vi "文件保存循环.vi"(8 "错误输入（无错误）":errorcluster, 10 "结束位队列":refnum<queue>, 11 "队列输入":refnum<queue>) -> (3 "总波形图表":waveform(i32)[](graph))   [LabVIEW 2020]
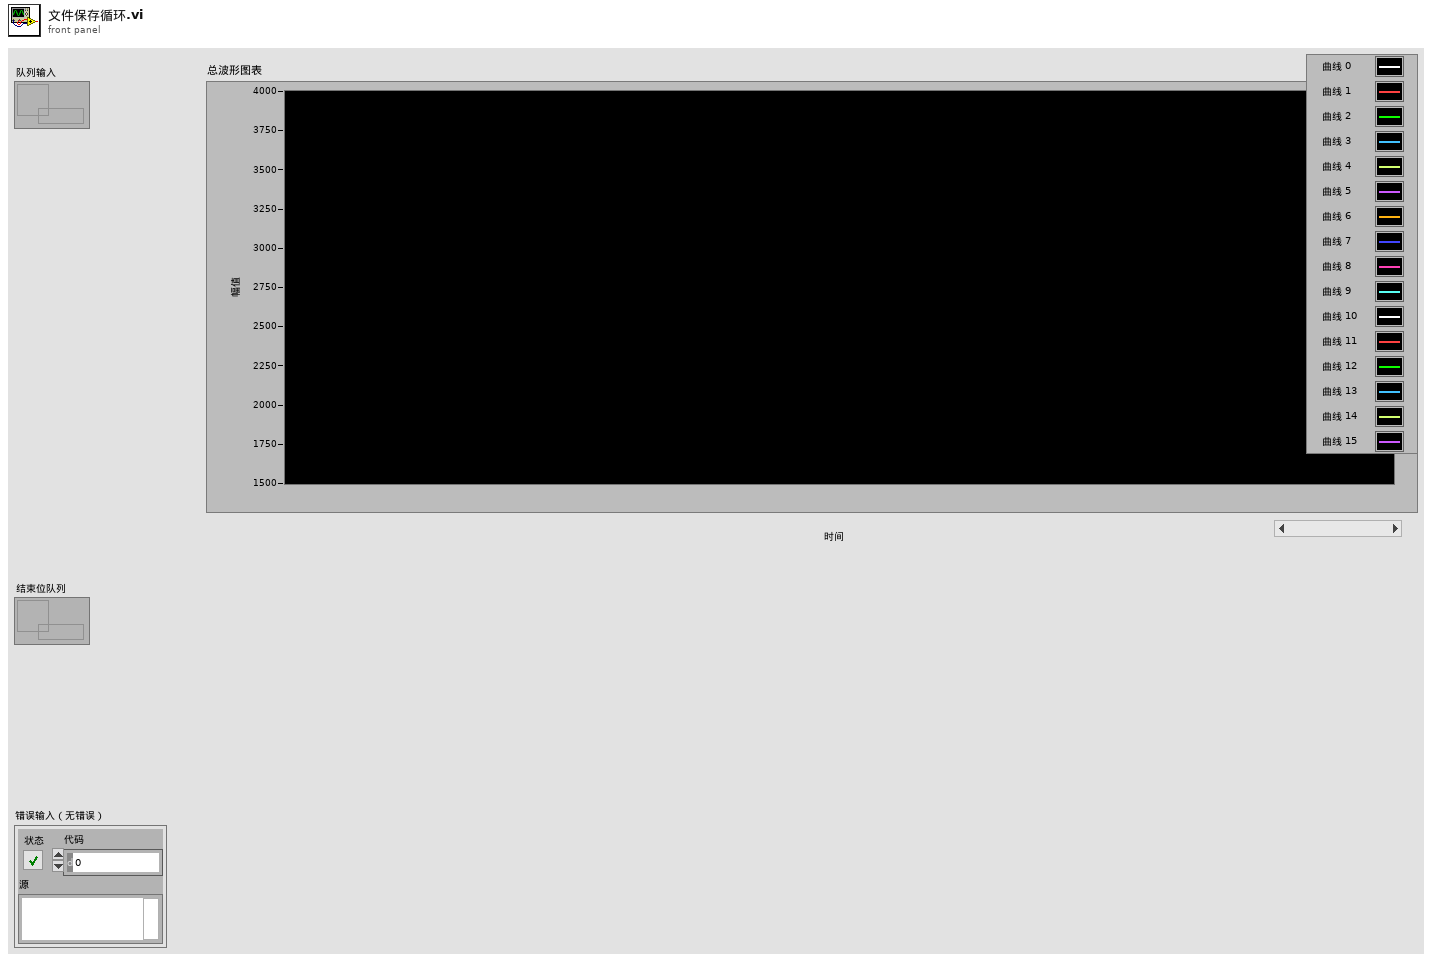
[diagram p1: front panel]
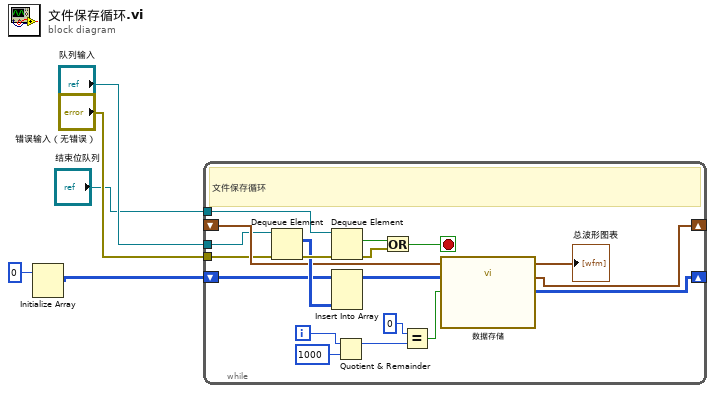
[diagram p0: block diagram]
diagram:
  n1 = Initialize Array(0) -> (w1:i32[][])  [unwired: 2 in]
  n2 = while {
    tunnel: "结束位队列" -> [w22]
    shift-right: [w11] -> _
    shift-left: w1 -> [w18]
    shift-right: [w10] -> _
    shift-left: _ -> [w9]
    tunnel: "错误输入（无错误）" -> [w7]
    tunnel: "队列输入" -> [w6]
    i -> [w17]
    stop <- w24 stop-if-true
    # "文件保存循环"
    n3 = Dequeue Element(queue=w6, error in (no error)=w7) -> (element=w19:i32[][], error out=w23:errorcluster)  [unwired: 1 in, 2 out]
    n4 = Dequeue Element(queue=w22, error in (no error)=w23) -> (element=w21:bool, error out=w20:errorcluster)  [unwired: 1 in, 2 out]
    n5 = Insert Into Array(array=w18, new element=w19) -> (w12:i32[][])  [unwired: 2 in]
    n6 = Quotient & Remainder(x=w17, y=1000) -> (x-y*floor(x/y)=w14:i32)  [unwired: 1 out]
    n7 = Or(x=w21, y=w20) -> (x .or. y?=w24:bool)
    n8 = Equal?(x=0, y=w14) -> (x = y?=w13:bool)
    n9 = call "数据存储.vi"("数据存储标志位"=w13, "数据输入"=w12, "上一时刻时间"=w9) -> ("初始化缓存"=w11:i32[][], "当前时间"=w10:timestamp, "波形图表 6"=→"总波形图表":waveform(i32)[])  [unwired: 6 in]
  }
